vi "DAQ error handler.vi"() -> ()   [LabVIEW 2018]
panel:
  in  "error in":errorcluster
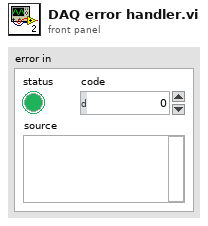
[diagram p1: front panel]
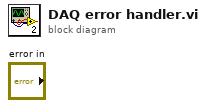
[diagram p0: block diagram]
diagram:
